vi "ArdnoRemoveAir.vi"(7 "ProgramSingleMultiring":u16, 8 "error in (no error)":errorcluster, 9 "ValveReagent":T7(ring), 11 "LINX Resource":T1) -> (0 "error out":errorcluster, 4 "ValveStates":bool[](array[boolean]))   [LabVIEW 2018, in "Arduino.lvlib"]
uses:
  Arduino.lvlib
  <vilib>/MakerHub/LINX/Private/Type Defs/LINX Ref.ctl
  <vilib>/MakerHub/LINX/Private/Type Defs/Platform.ctl
  <vilib>/MakerHub/LINX/Private/Type Defs/Interface.ctl
  <vilib>/MakerHub/LINX/Private/Device/Type Defs/LINX Device Config.ctl
  <vilib>/MakerHub/LINX/Private/Device/Type Defs/TCP Config.ctl
  <vilib>/MakerHub/LINX/Private/Device/Type Defs/Channels.ctl
  <vilib>/MakerHub/LINX/Public/Peripherals/Digital/Digital Write N Chans.vi
  <vilib>/MakerHub/LINX/Private/Local IO/LinxDigitalWrite.vi
  <vilib>/MakerHub/LINX/Public/Utilities/Check Channel.vi
  <vilib>/MakerHub/LINX/Private/Utilties/Generate Error.vi
  <vilib>/MakerHub/LINX/LMH-LINX.lvlib
  <vilib>/MakerHub/LINX/Private/Device/Device.lvlib
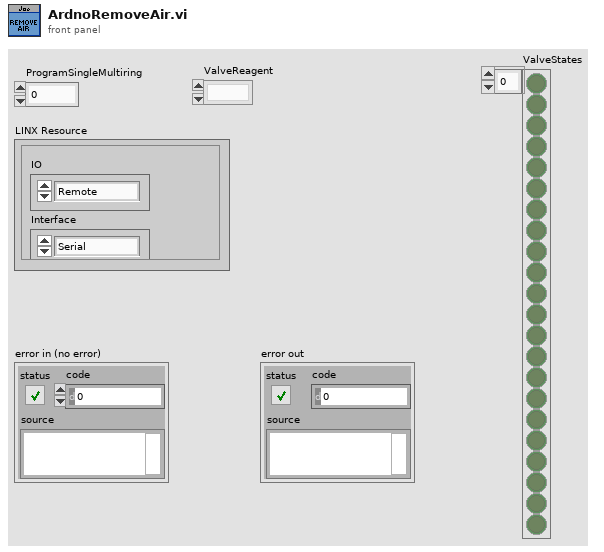
[diagram p1: front panel]
types:
  T1 = typedef "LMH-LINX.lvlib/LINX Ref.ctl" = cluster{"IO":T2, "Interface":T3, "LINX Device Config":T4}
  T2 = typedef "LMH-LINX.lvlib/Platform.ctl" = enum16{"Remote", "Local"}
  T3 = typedef "LMH-LINX.lvlib/Interface.ctl" = enum16{"Serial", "TCP"}
  T4 = typedef "LMH-LINX.lvlib/Device.lvlib/LINX Device Config.ctl" = cluster{"Interface":T3, "COM Port":refnum<visa-resource-name>, "TCP Configuration":T5, "Device Family":u8, "Device ID":u8, "Device Name":string, "TCP Ref":refnum<k5>, "Channels":T6}
  T5 = typedef "LMH-LINX.lvlib/Device.lvlib/TCP Config.ctl" = cluster{"IP Address":string, "Port":u16}
  T6 = typedef "LMH-LINX.lvlib/Channels.ctl" = cluster{"DI":u8[], "DO":u8[], "AI":u8[], "AO":u8[], "PWM":u8[], "QE":u8[], "UART":u8[], "I2C 2":u8[], "SPI":u8[], "CAN":u8[], "Servo":u8[], "AI Ref (V)":dbl, "AI Resolution (Bits)":u8, "AO Ref (V)":dbl, "AO Resolution (Bits)":u8}
  T7 = enum8{"", "1", "2", "3", "4", "5", "6", "7", "8", "9"}
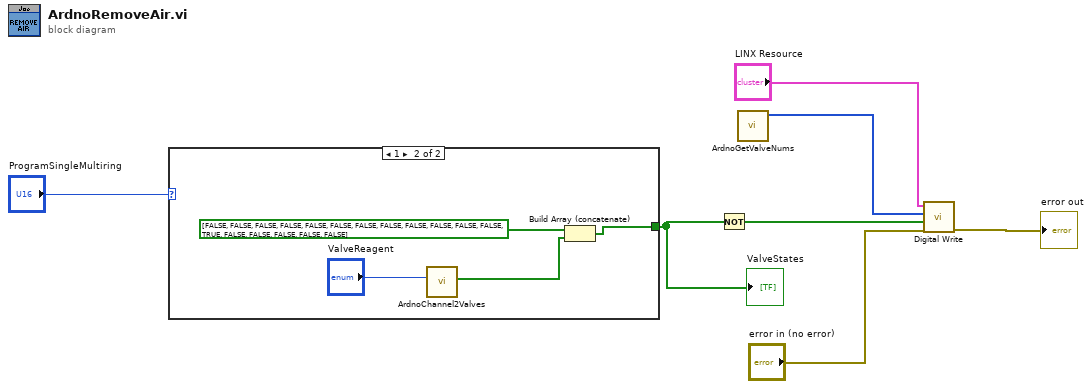
[diagram p0: block diagram]
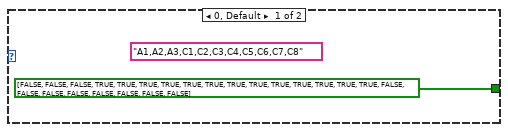
[diagram p2: hidden frame]
diagram:
  n1 = case shown="1" "ProgramSingleMultiring" {
    tunnel: [bool[] [FALSE, FALSE, FALSE, TRUE, TRUE, TRUE, TRUE, TRUE, TRUE, TRUE, TRUE, TRUE, TRUE, TRUE, TRUE, TRUE, FALSE, FALSE, FALSE, FALSE, FALSE, FALSE, FALSE, FALSE] w11] -> w4
    frame 0, Default {
      (unwired) "A1,A2,A3,C1,C2,C3,C4,C5,C6,C7,C8" ("Valve (A1-C8),\n comma separated")
    }
    frame 1 {
      n2 = call "ArdnoChannel2Valves.vi"("Reagent"="ValveReagent") -> ("Valve State"=w10:bool[])  [unwired: 9 in]
      n3 = Build Array (concatenate)(bool[] [FALSE, FALSE, FALSE, FALSE, FALSE, FALSE, FALSE, FALSE, FALSE, FALSE, FALSE, FALSE, TRUE, FALSE, FALSE, FALSE, FALSE, FALSE], w10) -> (w11:bool[])
    }
  }
  "ValveStates" <- w4
  n4 = Not(x=w4) -> (.not. x?=w1:bool[])
  n5 = call "ArdnoGetValveNums.vi"() -> ("Array"=w2:i32[])  [unwired: 11 in]
  n6 = call-poly <vilib>:"Digital Write.vi"("Error In"="error in (no error)", "Values"=w1, "DO Channels"=w2, "LINX Resource"="LINX Resource") -> ("Error Out"=→"error out":errorcluster)  [unwired: 6 in, 1 out]
